vi "Cleanup.vi"(8 "error in (no error)":errorcluster, 11 "VMR Server in":refnum<class "VMR Server.lvclass">) -> (0 "error out":errorcluster)   [LabVIEW 2022 SP3, in "VMR Server.lvlib" / "VMR Server.lvclass"]
uses:
  VMR Server.lvclass
  VMR Server.lvclass/VMR Server.ctl
  <vilib>/ActorFramework/Stop Msg/Stop Msg.lvclass
  <vilib>/IlluminatedG/IG HTTP Server/HTTP Server/Server/Server.lvclass
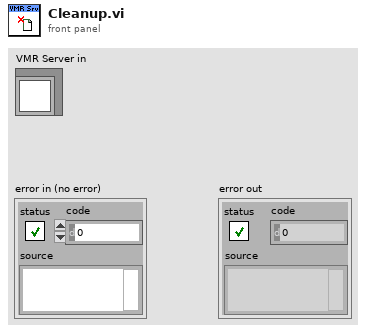
[diagram p1: front panel]
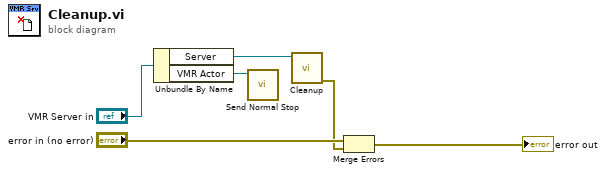
[diagram p0: block diagram]
diagram:
  n1 = Unbundle By Name("VMR Server in") -> ("Server"=w3:refnum<class "Server.lvclass">, "VMR Actor"=w4:refnum<class "Message Enqueuer.lvclass">)
  n2 = call <vilib>:"Send Normal Stop.vi"("Message Enqueuer"=w4) -> ()  [unwired: 10 in, 1 out]
  n3 = call <vilib>:"Cleanup.vi"("Server in"=w3) -> ("error out"=w1:errorcluster)  [unwired: 10 in]
  n4 = Merge Errors("error in (no error)", w1) -> (→"error out":errorcluster)
